vi "Global CN Config.vi"(8 "error in (no error)":errorcluster, 9 "Mode":enum16{"Init", "Read", "Write"}(ring), 10 "CN Config":T1[](array[typedef]), 11 "Path":path) -> (0 "error out":errorcluster, 3 "CN Config out":T1[](array[typedef]))   [LabVIEW 2014]
uses:
  Type'def/CN Config Ctr.ctl
  <vilib>/Utility/xml.llb/Read From XML File(string).vi
  <vilib>/Utility/xml.llb/Write to XML File(string).vi
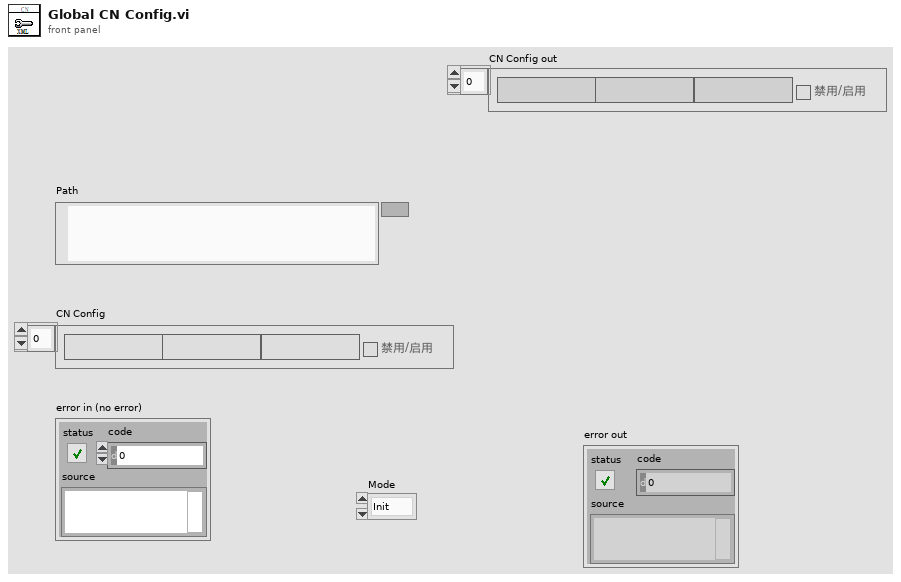
[diagram p1: front panel]
types:
  T1 = typedef "CN Config Ctr.ctl" = cluster{"Model":string, "Pic_Name":string, "CarName":string, "En/Disable":bool}
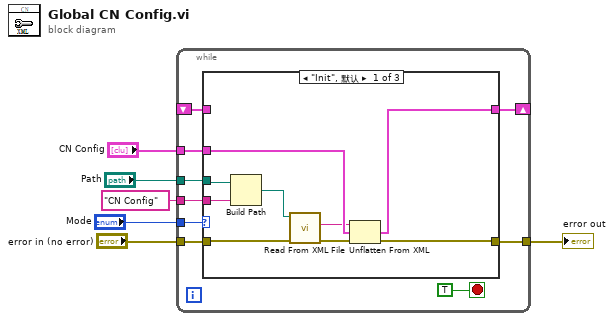
[diagram p0: block diagram]
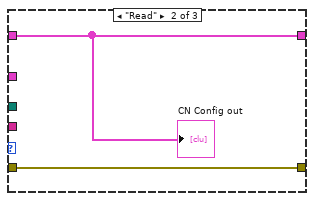
[diagram p2: hidden frame]
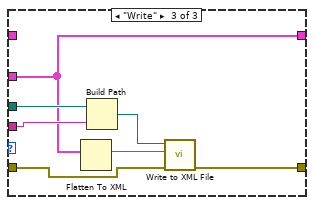
[diagram p3: hidden frame]
diagram:
  n1 = while {
    tunnel: "Mode" -> [w14]
    tunnel: "CN Config" -> [w13]
    tunnel: "error in (no error)" -> [w12]
    tunnel: "Path" -> [w11]
    tunnel: [w10] -> w2
    shift-right: [w9] -> _
    shift-left: _ -> [w7]
    tunnel: "CN Config" -> [w8]
    stop <- TRUE stop-if-true
    n2 = case shown="\"Init\", 默认" w14 {
      tunnel: w13 -> [w17 _ w29]
      tunnel: w12 -> [w24 w25 w28]
      tunnel: w11 -> [w23 _ w32]
      tunnel: [w19 w25 w33] -> w10
      tunnel: [w18 w26 w29] -> w9
      tunnel: w8 -> [w22 _ w30]
      tunnel: w7 -> [_ w26 _]
      frame "Init", Default {
        n3 = Build Path(base path=w23, name or relative path=w22) -> (appended path=w21:path)
        n4 = call-poly <vilib>:"Read From XML File.vi"("error in (no error)"=w24, "XML File Path"=w21) -> ("error out"=w20:errorcluster, "XML Elements"=w16:string)  [unwired: 7 in, 1 out]
        n5 = Unflatten From XML(xml string=w16, type=w17, error in (no error)=w20) -> (value=w18:T1[], error out=w19:errorcluster)
      }
      frame "Read" {
        "CN Config out" <- w26
      }
      frame "Write" {
        n6 = Flatten To XML(anything=w29) -> (xml string=w27:string)
        n7 = Build Path(base path=w32, name or relative path=w30) -> (appended path=w31:path)
        n8 = call-poly <vilib>:"Write to XML File.vi"("error in (no error)"=w28, "XML Input"=w27, "XML File Path"=w31) -> ("error out"=w33:errorcluster)  [unwired: 6 in, 2 out]
      }
    }
  }
  "error out" <- w2
